vi "validate line configuration.vi"(7 "io configuration":refnum<class "io configuration.lvclass">, 11 "line in":T1) -> (1 "valid?":bool, 2 "errors":string, 3 "line out":T1)   [LabVIEW 2017, in "io editor node.lvclass"]
uses:
  io editor node.lvclass
  table line.ctl
  <vilib>/NI/Tag Bus Module Framework/channel/TBM channel.lvclass
  C:/Program Files (x86)/National Instruments/LabVIEW 2017/vi.lib/NI/Tag Bus/tag/tag descriptor.lvclass
  configuration/io configuration.lvclass
  <vilib>/NI/Tag Bus/tag/tag descriptor.lvclass/tag descriptor.ctl
  <vilib>/NI/Tag Bus/tag/read tag name.vi
  <vilib>/NI/Tag Bus/tag/read data type.vi
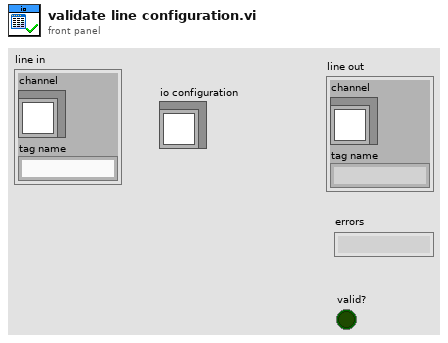
[diagram p1: front panel]
types:
  T1 = typedef "io editor node.lvclass/table line.ctl" = cluster{"channel":refnum<class "TBM channel.lvclass">, "tag name":string}
  T2 = typedef "tag bus.lvlib/tag descriptor.lvclass/Data Type.ctl" = enum16{"Double", "Single", "I64", "I32", "I16", "I8", "U64", "U32", "U16", "U8", "Boolean", "String", "Array of Double", "Array of Single", "Array of I64", "Array of I32", "Array of I16", "Array of I8", "Array of U64", "Array of U32", "Array of U16", "Array of U8", "Array of Boolean", "Array of String"}
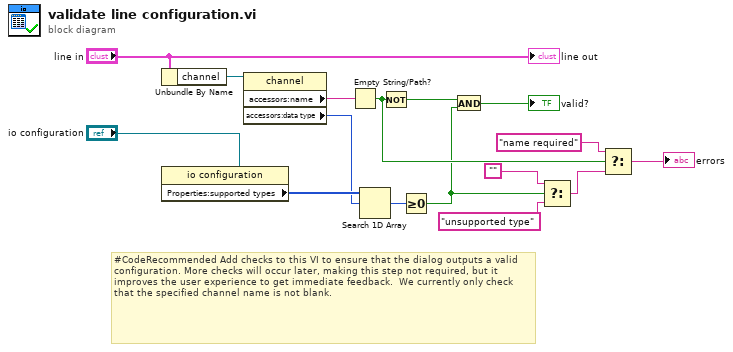
[diagram p0: block diagram]
diagram:
  # "#CodeRecommended Add checks to this VI to ensure that the dialog outputs a valid configuration. More checks will occur later, making this step not required, but it improves the user experience to get immediate feedback.  We currently only check that the specified channel name is not blank."
  n1 = Unbundle By Name("line in") -> ("channel"=w15:refnum<class "TBM channel.lvclass">)
  n2 = property class="io configuration"(reference="io configuration") -> ("Properties:supported types"=w12:T2[])  [unwired: 1 in, 2 out]
  n3 = property class="channel"(reference=w15) -> ("accessors:name"=w14:string, "accessors:data type"=w11:T2)  [unwired: 1 in, 2 out]
  n4 = Empty String/Path?(string/path=w14) -> (empty?=w8:bool)
  n5 = Search 1D Array(1D array=w12, element=w11) -> (index of element=w9:i32)  [unwired: 1 in]
  n6 = Not(x=w8) -> (.not. x?=w13:bool)
  n7 = Greater Or Equal To 0?(x=w9) -> (x >= 0?=w5:bool)
  n8 = And(x=w13, y=w5) -> (x .and. y?=→"valid?":bool)
  n9 = Select(t="", s=w5, f="unsupported type") -> (s? t:f=w3:string)
  n10 = Select(t="name required", s=w8, f=w3) -> (s? t:f=→"errors":string)
  "line out" <- "line in"
